vi "Initialize MeasurementLink Session.vi"(7 "remote connection options":T2, 8 "error in":errorcluster, 9 "initialize and close session behavior":T1, 10 "session initialization parameters":T3, 11 "session factory in":refnum<class "Session Factory.lvclass">) -> (0 "error out":errorcluster, 2 "session out":variant, 3 "session factory out":refnum<class "Session Factory.lvclass">)   [LabVIEW 2020, in "MeasurementLink VISA.lvlib" / "Session Factory.lvclass"]
uses:
  Session Factory.lvclass
  MeasurementLink Instrument/ISession Factory/Session Initialization Parameters.ctl
  MeasurementLink Instrument/ISession Factory/Remote Connection Options.ctl
  MeasurementLink Instrument/ISession Factory/Initialize and Close Session Behavior.ctl
  Session Factory.lvclass/Session Factory.ctl
  MeasurementLink Instrument/ISession Factory/ISession Factory.lvclass
  <vilib>/NI-VISA/VISA Open for gRPC Session.vi
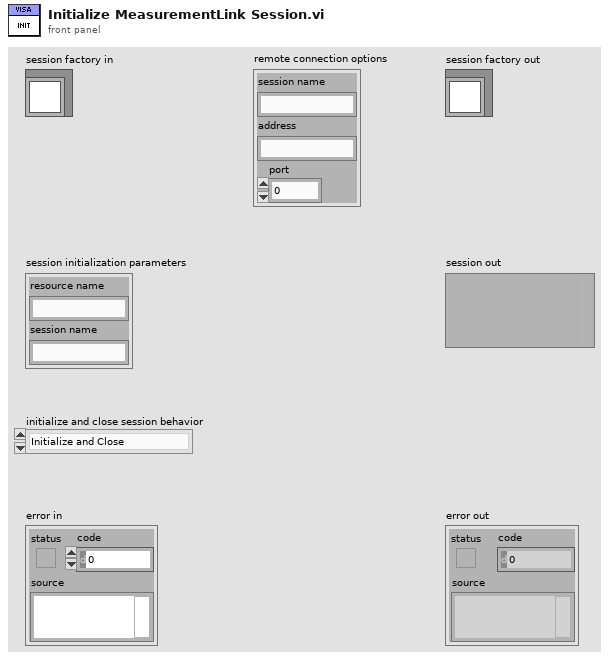
[diagram p1: front panel]
types:
  T1 = typedef "MeasurementLink Instrument.lvlib/ISession Factory.lvclass/Initialize and Close Session Behavior.ctl" = enum16{"Initialize and Close", "Attach and Detach", "Initialize and Detach", "Attach and Close"}
  T2 = typedef "MeasurementLink Instrument.lvlib/ISession Factory.lvclass/Remote Connection Options.ctl" = cluster{"session name":string, "address":string, "port":u32}
  T3 = typedef "MeasurementLink Instrument.lvlib/ISession Factory.lvclass/Session Initialization Parameters.ctl" = cluster{"resource name":string, "session name":string}
  T4 = typedef "VISA Open Access Mode.ctl" = u32
  T5 = typedef "VISA gRPC Open Close Behavior.ctl" = enum16{"Auto", "Initialize and Close", "Attach and Detach", "Initialize and Detach", "Attach and Close"}
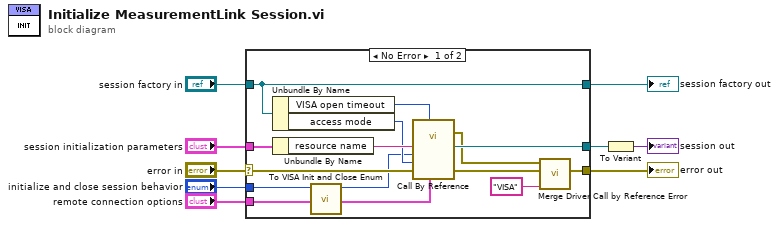
[diagram p0: block diagram]
diagram:
  n1 = case shown="No Error" "error in" {
    selector: "error in" -> [w21 w24]
    tunnel: [w16 w24] -> w8
    tunnel: "session factory in" -> [w14 w25]
    tunnel: [w14 w25] -> w6
    tunnel: "remote connection options" -> [w23 _]
    tunnel: "session initialization parameters" -> [w20 _]
    tunnel: [w22 _] -> w3
    tunnel: "initialize and close session behavior" -> [w11 _]
    frame No Error {
      n2 = Unbundle By Name(w14) -> ("VISA open timeout"=w12:u32, "access mode"=w13:T4)
      n3 = Unbundle By Name(w20) -> ("resource name"=w19:string)
      n4 = call "To VISA Init and Close Enum.vi"("factory init and close behavior"=w11) -> ("visa init and close behavior"=w10:T5)  [unwired: 10 in]
      n5 = call-by-ref "?"("gRPC Options"=w23, "VISA Open Timeout (0)"=w12, "error in (no error)"=w21, "Access Mode"=w13, "Open/Close Behavior"=w10, "VISA resource name"=w19) -> (error out=w17:errorcluster, 0:"error out"=w18:errorcluster, "VISA resource name out"=w22:refnum<visa-resource-name>)  [unwired: 6 in, 1 out]
      n6 = call "Merge Driver Call by Reference Error.vi"("driver name"="VISA", "called vi error"=w18, "call by ref error"=w17) -> ("error out"=w16:errorcluster)  [unwired: 8 in]
    }
    frame Error {
    }
  }
  "error out" <- w8
  "session factory out" <- w6
  n7 = To Variant(anything=w3) -> (Variant=→"session out":variant)
